vi "domeADB_logEvent_DriveDisabled.vi"(8 "error in (no error)":errorcluster, 11 "logevent_DriveDisabled_Ctl":T1) -> (0 "error out":errorcluster, 2 "function return":i32, 3 "logevent_DriveDisabled_Ctl out":T1)   [LabVIEW 2016, in "SALLV_domeADB.lvlib"]
doc: "int domeADB_shm_logEvent_DriveDisabledLV(domeADB_logevent_DriveDisabledLV *logevent_DriveDisabled_Ctl );"
uses:
  SALLV_domeADB.lvlib
  DataTypes/logevent_DriveDisabled.ctl
  SALLV_domeADB.so
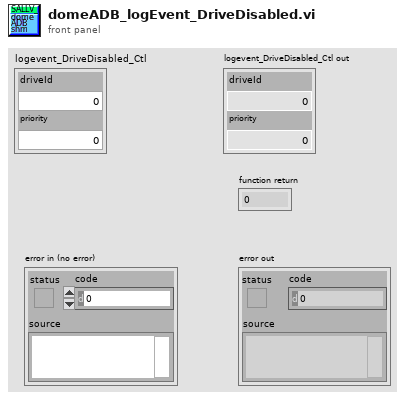
[diagram p1: front panel]
types:
  T1 = typedef "SALLV_domeADB.lvlib/logevent_DriveDisabled.ctl" = cluster{"driveId":i32, "priority":i32}
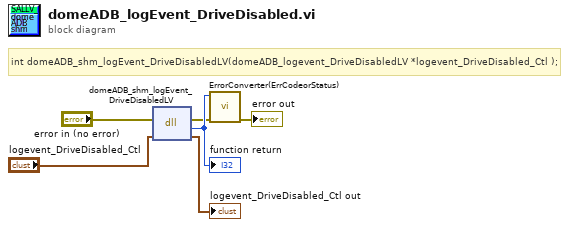
[diagram p0: block diagram]
diagram:
  # "int domeADB_shm_logEvent_DriveDisabledLV(domeADB_logevent_DriveDisabledLV *logevent_DriveDisabled_Ctl );"
  n1 = dll-call lib="home/andres/Desktop/SALLV_domeADB/SALLV_domeADB.*" fn="domeADB_shm_logEvent_DriveDisabledLV"(error in="error in (no error)", "logevent_DriveDisabled_Ctl"="logevent_DriveDisabled_Ctl") -> (error out=w2:errorcluster, w6:i32, "logevent_DriveDisabled_Ctl"=→"logevent_DriveDisabled_Ctl out":T1)  [unwired: 2 in, 1 out]
  "function return" <- w6
  n2 = call "ErrorConverter(ErrCodeorStatus).vi"("error in (no error)"=w2, "error code"=w6) -> ("error out"=→"error out":errorcluster)  [unwired: 9 in]
